vi "MAD_Result.vi"(8 "error in":errorcluster, 10 "ResultArray":string[](array[string]), 11 "XLS in":refnum<class "XLS.lvclass">=refnum) -> (0 "error out":errorcluster, 3 "XLS out":refnum<class "XLS.lvclass">)   [LabVIEW 2017, in "Report_lib.lvlib" / "XLS.lvclass"]
uses:
  XLS.lvclass
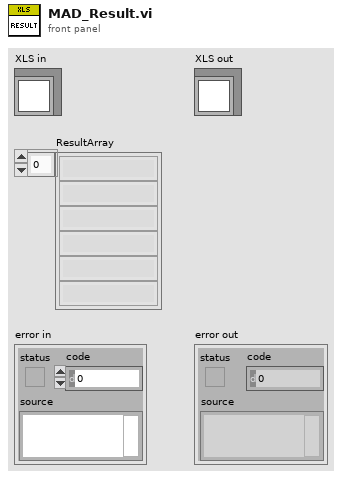
[diagram p1: front panel]
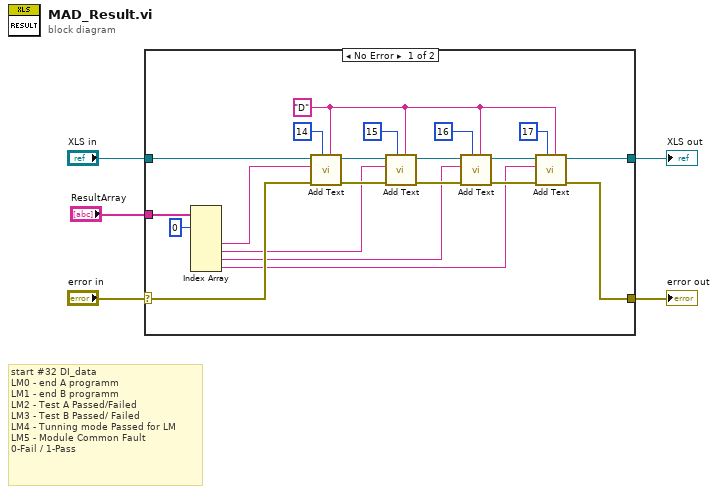
[diagram p0: block diagram]
diagram:
  # "start #32 DI_data\nLM0 - end A programm \nLM1 - end B programm\nLM2 - Test A Passed/Failed\nLM3 - Test B Passed/ Failed\nLM4 - Tunning mode Passed for LM\nLM5 - Module Common Fault\n0-Fail / 1-Pass"
  n1 = case shown="No Error" "error in" {
    selector: "error in" -> [w20 w28]
    tunnel: [w16 w28] -> w4
    tunnel: [w11 w27] -> w2
    tunnel: "XLS in" -> [w15 w27]
    tunnel: "ResultArray" -> [w25 _]
    frame No Error {
      w10 = "D" ("Adr")
      n2 = Index Array(array=w25, index #1=0 ("index")) -> (element #3=w9:string, element #4=w8:string, element #5=w7:string, element #6=w6:string)  [unwired: 5 in, 2 out]
      n3 = call "Add Text.vi"("Adr"=w10, "Index"=14, "error in"=w20, "text"=w9, "XLS in"=w15) -> ("error out"=w19:errorcluster, "XLS out"=w14:refnum<class "XLS.lvclass">)  [unwired: 5 in]
      n4 = call "Add Text.vi"("Adr"=w10, "Index"=15, "error in"=w19, "text"=w8, "XLS in"=w14) -> ("error out"=w18:errorcluster, "XLS out"=w13:refnum<class "XLS.lvclass">)  [unwired: 5 in]
      n5 = call "Add Text.vi"("Adr"=w10, "Index"=16, "error in"=w18, "text"=w7, "XLS in"=w13) -> ("error out"=w17:errorcluster, "XLS out"=w12:refnum<class "XLS.lvclass">)  [unwired: 5 in]
      n6 = call "Add Text.vi"("Adr"=w10, "Index"=17, "error in"=w17, "text"=w6, "XLS in"=w12) -> ("error out"=w16:errorcluster, "XLS out"=w11:refnum<class "XLS.lvclass">)  [unwired: 5 in]
    }
    frame Error {
    }
  }
  "error out" <- w4
  "XLS out" <- w2
